vi "Pump Status.vi"(8 "error in (no error)":errorcluster, 11 "SSI PR Settings":T1) -> (0 "error out":errorcluster, 1 "Connection Error":bool, 2 "Pump On?":enum16{"Off", "On", "Not Initialized"}(ring), 3 "SSI PR Settings":T1, 4 "Pressure":dbl format="%#_13g", 5 "Flow":dbl)   [LabVIEW 2018, in "SSI PR Pump.lvlib"]
uses:
  SSI PR Pump.lvlib
  SSI PR Settings Cluster.ctl
  <vilib>/regexp/Match Regular Expression.xnode
panel:
  out "after match":string
  out "read buffer 3":string
  out "whole match":string
  out "before match":string
  out "read buffer 2":string
  out "read buffer":string
  out "Flow 2":string
  out "Pressure":string
  out "0":string
  out "Stop/Start":string
  out "0":string
  out "p_units":string
  out "LPL":string
  out "UPL":string
  out "Flow":string
  out "OK":string
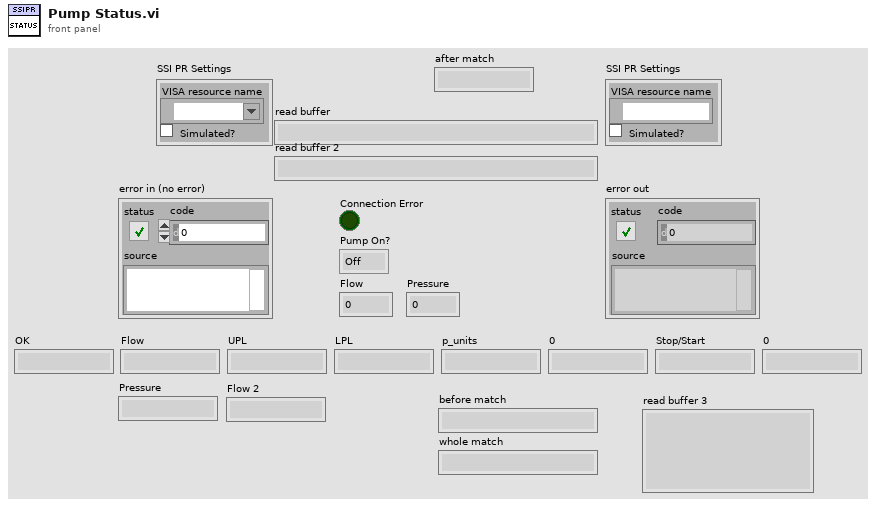
[diagram p1: front panel]
types:
  T1 = typedef "SSI PR Pump.lvlib/SSI PR Settings Cluster.ctl" = cluster{"VISA resource name":refnum<visa-resource-name>, "Simulated?":bool}
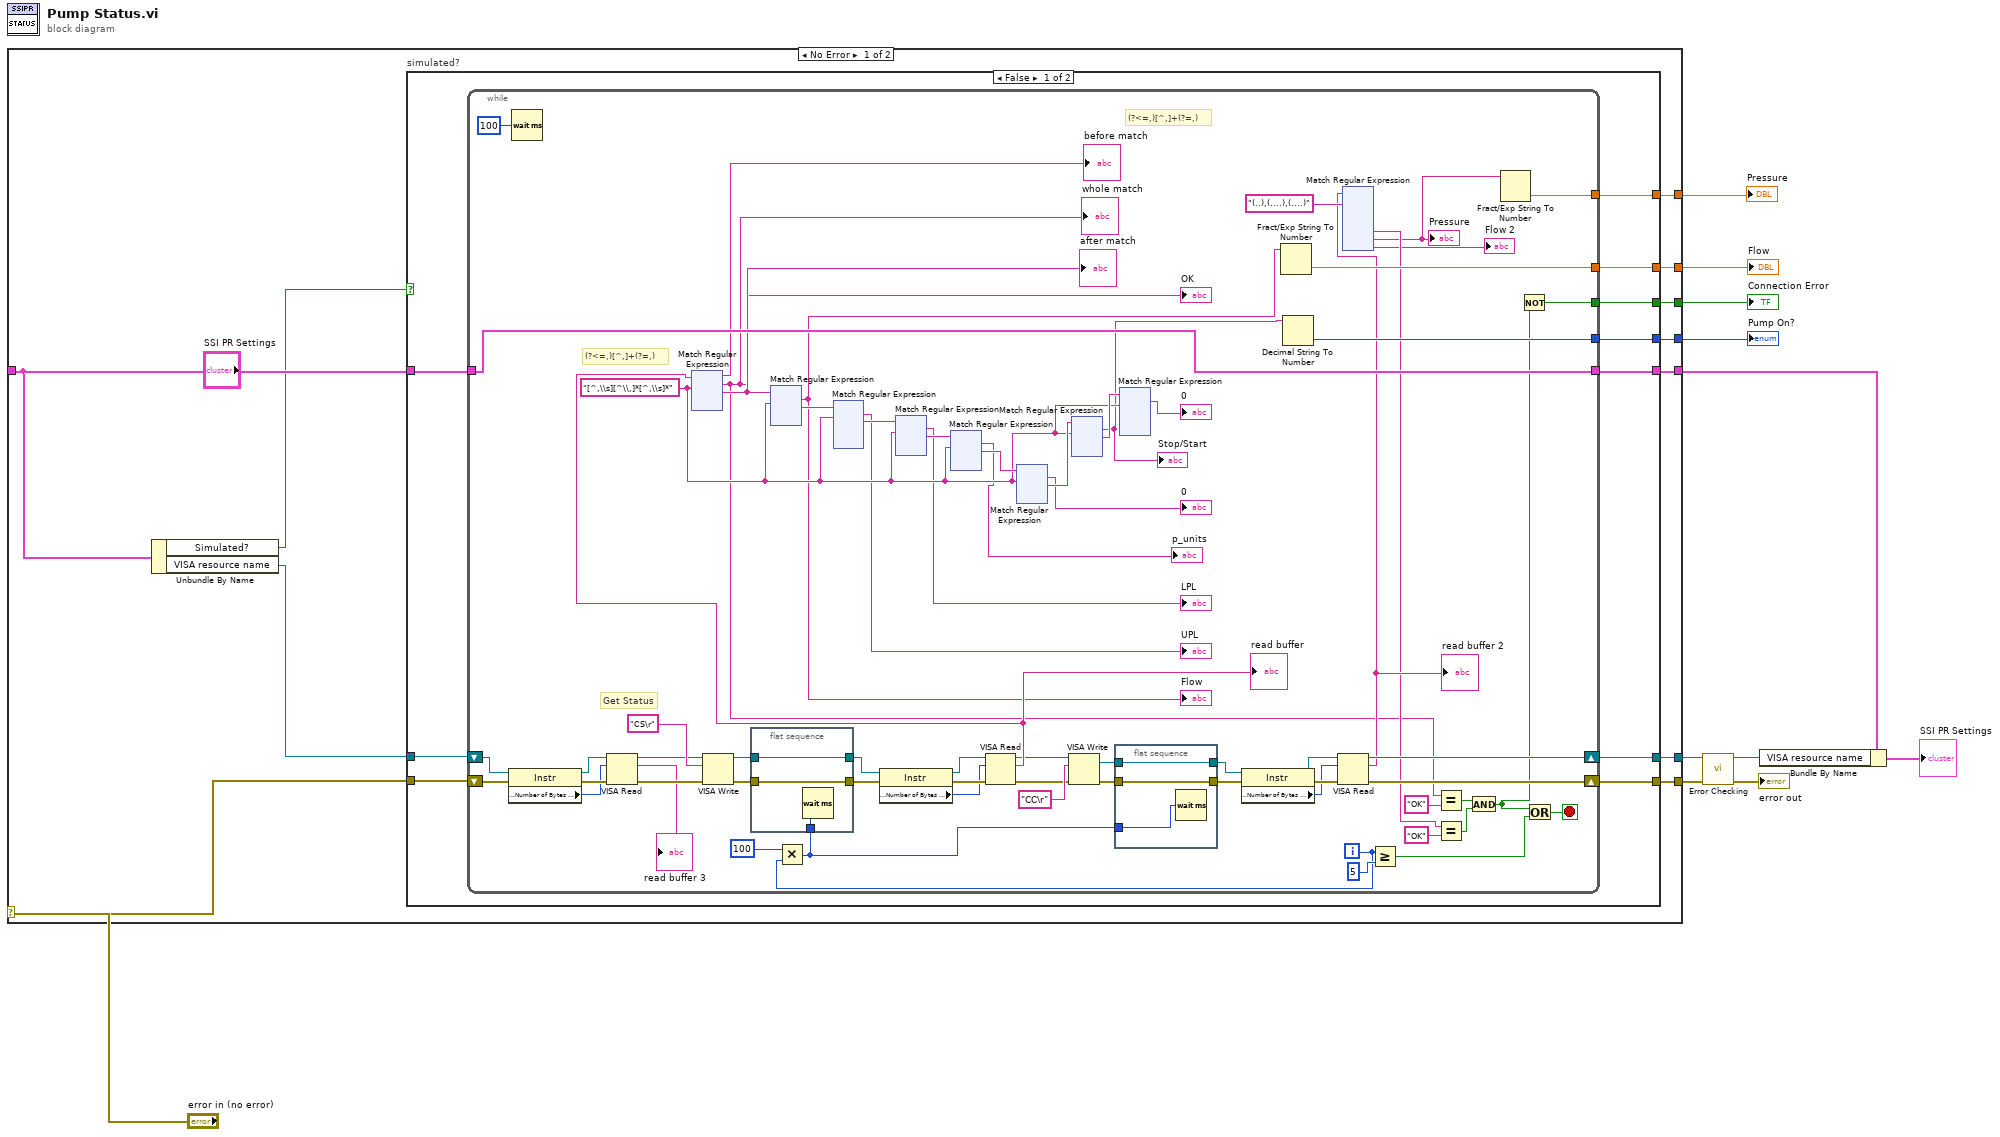
[diagram p0: block diagram]
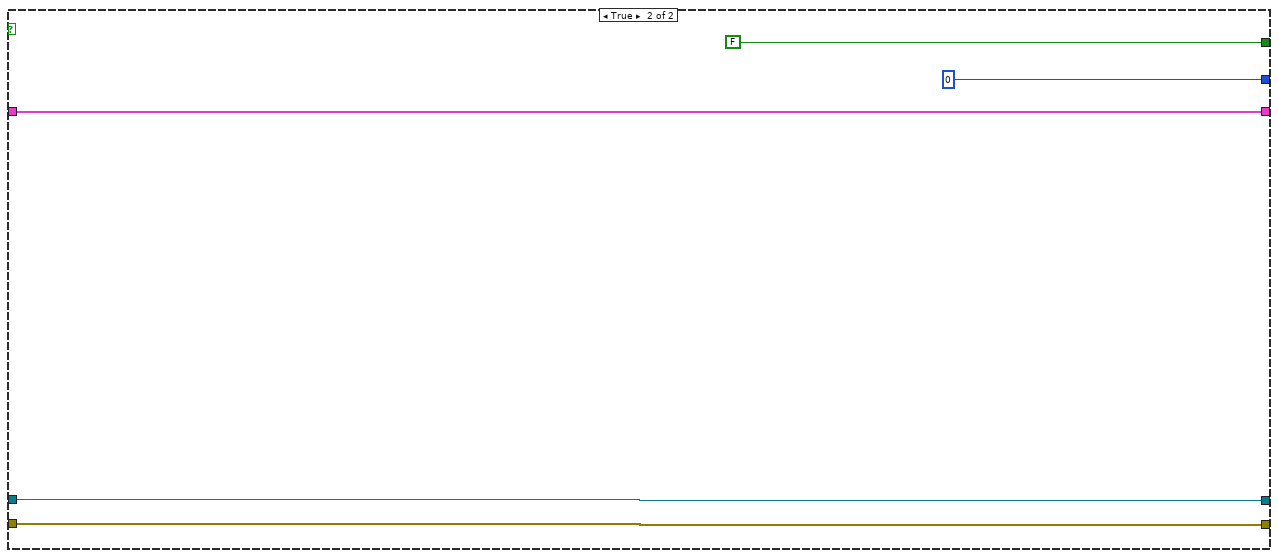
[diagram p2: hidden frame]
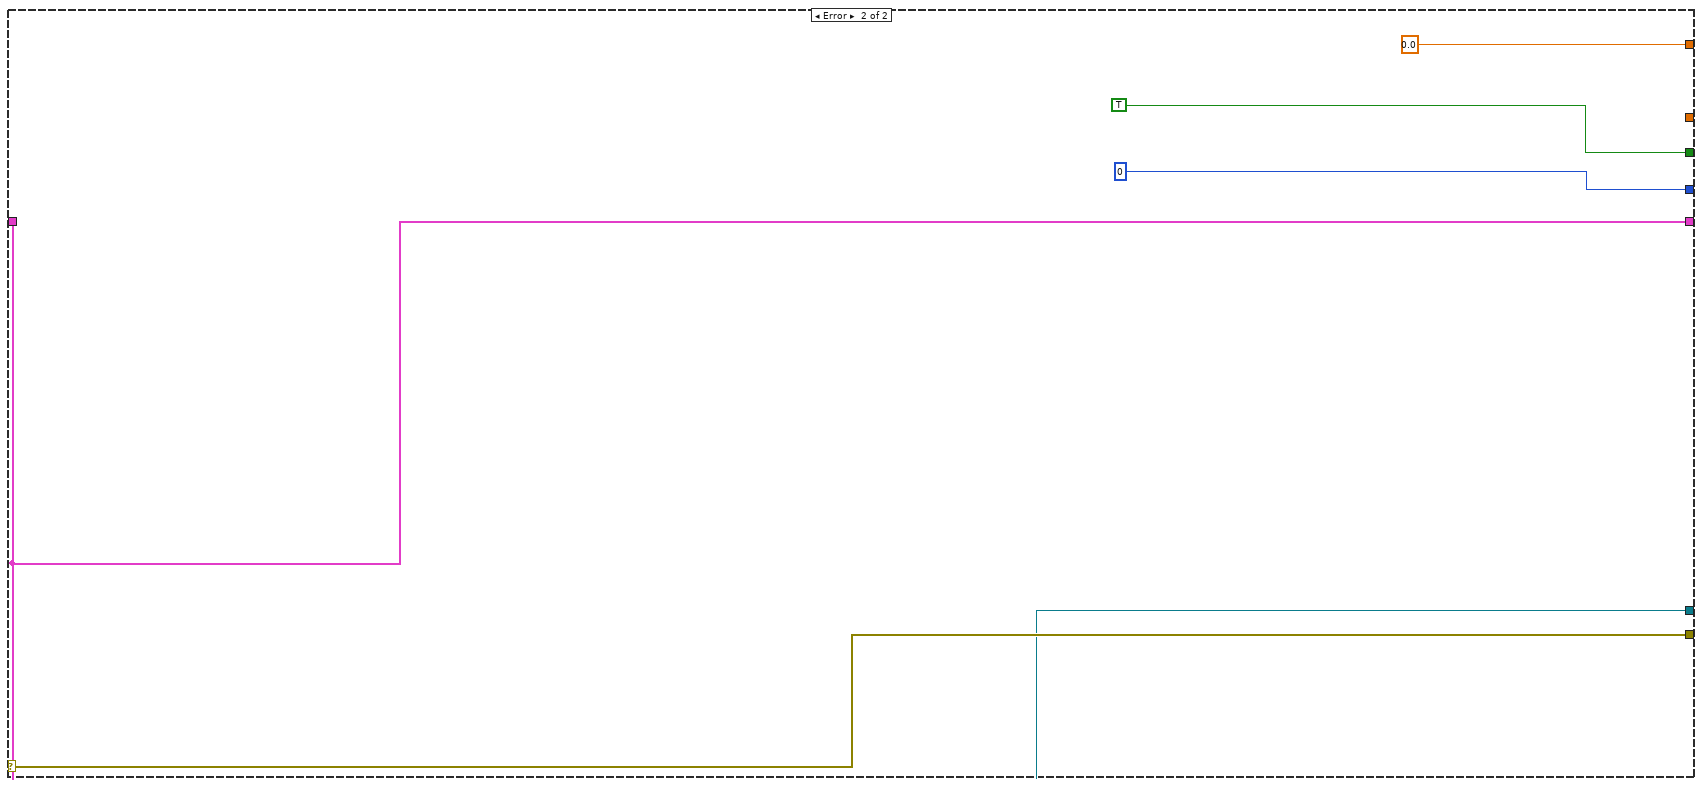
[diagram p3: hidden frame]
diagram:
  n1 = case shown="No Error" "error in (no error)" {
    selector: "error in (no error)" -> [w23 w1152]
    tunnel: [w19 w1151] -> w9
    tunnel: "SSI PR Settings" -> [w20 w1151]
    tunnel: [w22 w1150] -> w5
    tunnel: [w21 w1152] -> w6
    tunnel: [w16 TRUE] -> w4
    tunnel: [w15 0] -> w3
    tunnel: [w14 _] -> w2
    tunnel: [w13 0.0] -> w1
    frame No Error {
      n2 = Unbundle By Name(w20) -> ("Simulated?"=w17:bool, "VISA resource name"=w18:refnum<visa-resource-name>)
      n3 = case "simulated?" shown="False" w17 {
        tunnel: [w31 w1146] -> w22
        tunnel: w18 -> [w33 w1146]
        tunnel: w23 -> [w32 w1145]
        tunnel: [w30 w1145] -> w21
        tunnel: w20 -> [w29 w1144]
        tunnel: [w28 w1144] -> w19
        tunnel: [w27 FALSE] -> w16
        tunnel: [w26 0] -> w15
        tunnel: [w25 _] -> w14
        tunnel: [w24 _] -> w13
        frame False {
          n4 = while {
            shift-right: [w87] -> w31
            shift-left: w33 -> [w57]
            shift-right: [w86] -> w30
            shift-left: w32 -> [w56]
            tunnel: w29 -> [w101]
            tunnel: [w101] -> w28
            tunnel: [w93] -> w27
            tunnel: [w92] -> w26
            tunnel: [w91] -> w25
            tunnel: [w76] -> w24
            i -> [w35]
            stop <- w94 stop-if-true
            w45 = "[^,\\s][^\\,]*[^,\\s]*" ("regular expression")
            # "(?<=,)[^,]+(?=,)"
            # "(?<=,)[^,]+(?=,)"
            # "Get Status"
            n5 = property class="Instr"(reference=w57, error in=w56) -> (reference out=w59:refnum<visa-resource-name>, error out=w60:errorcluster, "Serial Settings:Number of Bytes at Serial Port"=w58:u32)
            n6 = Wait (ms)(milliseconds to wait=u32 100) -> ()  [unwired: 1 out]
            n7 = VISA Read(VISA resource name=w59, byte count=w58, error in (no error)=w60) -> (VISA resource name out=w55:refnum<visa-resource-name>, read buffer=→"read buffer 3":string, error out=w54:errorcluster)  [unwired: 1 out]
            n8 = VISA Write(VISA resource name=w55, write buffer="CS\r" ("string"), error in (no error)=w54) -> (VISA resource name out=w68:refnum<visa-resource-name>, error out=w70:errorcluster)  [unwired: 1 out]
            n9 = flat-sequence {
              tunnel: [w909] -> w71
              tunnel: w70 -> [w909]
              tunnel: [w908] -> w69
              tunnel: w68 -> [w908]
              tunnel: w34 -> [w907]
              frame #0 {
                n10 = Wait (ms)(milliseconds to wait=w907) -> ()  [unwired: 1 out]
              }
            }
            n11 = Multiply(x=u32 100 ("milliseconds to wait"), y=w35) -> (x*y=w34:u32)
            n12 = property class="Instr"(reference=w69, error in=w71) -> (reference out=w67:refnum<visa-resource-name>, error out=w75:errorcluster, "Serial Settings:Number of Bytes at Serial Port"=w62:u32)
            n13 = VISA Read(VISA resource name=w67, byte count=w62, error in (no error)=w75) -> (VISA resource name out=w89:refnum<visa-resource-name>, read buffer=w98:string, error out=w88:errorcluster)  [unwired: 1 out]
            "read buffer" <- w98
            n14 = xnode "Match Regular Expression"("input string"=w98, "regular expression"=w45) -> ("before match"=→"before match":string, "whole match"=w44:string, "after match"=w52:string)  [unwired: 4 in, 2 out]
            "OK" <- w44
            "whole match" <- w44
            "after match" <- w52
            n15 = xnode "Match Regular Expression"("input string"=w52, "regular expression"=w45) -> ("whole match"=w43:string, "after match"=w51:string)  [unwired: 4 in, 3 out]
            "Flow" <- w43
            n16 = xnode "Match Regular Expression"("input string"=w51, "regular expression"=w45) -> ("whole match"=→"UPL":string, "after match"=w50:string)  [unwired: 4 in, 4 out]
            n17 = xnode "Match Regular Expression"("input string"=w50, "regular expression"=w45) -> ("whole match"=→"LPL":string, "after match"=w49:string)  [unwired: 4 in, 3 out]
            n18 = xnode "Match Regular Expression"("input string"=w49, "regular expression"=w45) -> ("whole match"=→"p_units":string, "after match"=w48:string)  [unwired: 4 in, 3 out]
            n19 = xnode "Match Regular Expression"("input string"=w48, "regular expression"=w45) -> ("whole match"=→"0":string, "after match"=w47:string)  [unwired: 4 in, 3 out]
            n20 = VISA Write(VISA resource name=w89, write buffer="CC\r" ("string"), error in (no error)=w88) -> (VISA resource name out=w65:refnum<visa-resource-name>, error out=w64:errorcluster)  [unwired: 1 out]
            n21 = xnode "Match Regular Expression"("input string"=w47, "regular expression"=w45) -> ("whole match"=w38:string, "after match"=w46:string)  [unwired: 4 in, 3 out]
            "Stop/Start" <- w38
            n22 = flat-sequence {
              tunnel: [w906] -> w66
              tunnel: w65 -> [w906]
              tunnel: w64 -> [w905]
              tunnel: [w905] -> w63
              tunnel: w34 -> [w904]
              frame #0 {
                n23 = Wait (ms)(milliseconds to wait=w904) -> ()  [unwired: 1 out]
              }
            }
            n24 = xnode "Match Regular Expression"("input string"=w46, "regular expression"=w45) -> ("whole match"=→"0":string)  [unwired: 4 in, 5 out]
            n25 = property class="Instr"(reference=w66, error in=w63) -> (reference out=w74:refnum<visa-resource-name>, error out=w73:errorcluster, "Serial Settings:Number of Bytes at Serial Port"=w72:u32)
            n26 = Fract/Exp String To Number(string=w43) -> (number=w91:dbl)  [unwired: 3 in, 1 out]
            n27 = Decimal String To Number(string=w38) -> (number=w92:i32)  [unwired: 2 in, 1 out]
            n28 = VISA Read(VISA resource name=w74, byte count=w72, error in (no error)=w73) -> (VISA resource name out=w87:refnum<visa-resource-name>, read buffer=w84:string, error out=w86:errorcluster)  [unwired: 1 out]
            "read buffer 2" <- w84
            n29 = xnode "Match Regular Expression"("input string"=w84, "regular expression"="(..),(....),(....)") -> ("submatch 1"=w82:string, "submatch 2"=w77:string, "submatch 3"=→"Flow 2":string)  [unwired: 4 in, 5 out]
            "Pressure" <- w77
            n30 = Greater Or Equal?(x=w35, y=5) -> (x >= y?=w95:bool)
            n31 = Equal?(x=w44, y="OK") -> (x = y?=w81:bool)
            n32 = Equal?(x=w82, y="OK") -> (x = y?=w80:bool)
            n33 = And(x=w81, y=w80) -> (x .and. y?=w79:bool)
            n34 = Fract/Exp String To Number(string=w77) -> (number=w76:dbl)  [unwired: 3 in, 1 out]
            n35 = Not(x=w79) -> (.not. x?=w93:bool)
            n36 = Or(x=w79, y=w95) -> (x .or. y?=w94:bool)
          }
        }
        frame True {
        }
      }
    }
    frame Error {
      n37 = Unbundle By Name(w1151) -> ("VISA resource name"=w1150:refnum<visa-resource-name>)
    }
  }
  "Connection Error" <- w4
  "Pump On?" <- w3
  "Flow" <- w2
  "Pressure" <- w1
  n38 = call "Error Checking.vi"("error in (no error)"=w6, "VISA resource name"=w5) -> ("error out"=→"error out":errorcluster, "VISA resource name"=w7:refnum<visa-resource-name>)  [unwired: 7 in, 1 out]
  n39 = Bundle By Name(cluster=w9, "VISA resource name"=w7) -> (→"SSI PR Settings":T1)
